vi "Configure System Mode.vi"(8 "error in (no error)":errorcluster, 10 "System Mode (0: Local)":i32(ring) items=["Local", "Remote", "Remote with Lock", "Voltage", "Current", "Dual"], 11 "VISA resource name":refnum<visa-resource-name>) -> (0 "error out":errorcluster, 3 "VISA resource name out":refnum<visa-resource-name>)   [LabVIEW 2018, in "XP Power PLS600.lvlib"]
doc: "Sets the Control Source of the power supply to the specified value. Control Sources include: Local control from the front panel of the instrument, Remote control over the SCPI interface with limited front panel functionality, Remote with Lock control over the SCPI interface with no front panel capability, Analog Voltage Control where the voltage setpoint is determined by the analog voltage input, Analog Current Control where the current setpoint is determined by the analog current input, or Dual Analog Control where the voltage and current setpoint are determined by their respective analog inputs."
uses:
  XP Power PLS600.lvlib
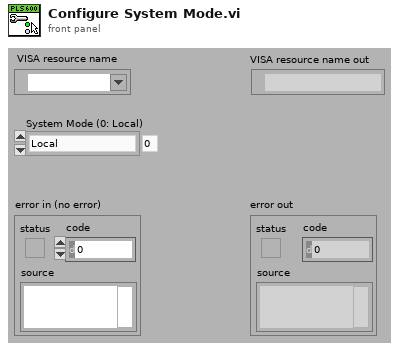
[diagram p1: front panel]
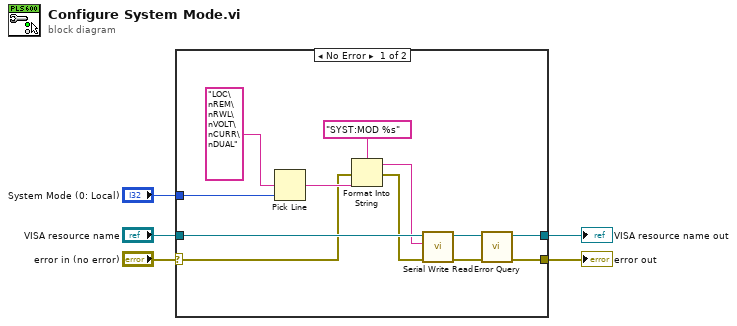
[diagram p0: block diagram]
diagram:
  n1 = case shown="No Error" "error in (no error)" {
    selector: "error in (no error)" -> [w8 w18]
    tunnel: "System Mode (0: Local)" -> [w16 _]
    tunnel: [w15 w19] -> w4
    tunnel: [w14 w18] -> w3
    tunnel: "VISA resource name" -> [w13 w19]
    frame No Error {
      n2 = Pick Line(multi-line string="LOC\nREM\nRWL\nVOLT\nCURR\nDUAL", line index=w16) -> (output string=w9:string)  [unwired: 1 in]
      n3 = Format Into String(format string="SYST:MOD %s" ("Command to Send"), error in=w8, w9) -> (resulting string=w6:string, error out=w7:errorcluster)  [unwired: 1 in]
      n4 = call "Serial Write Read.vi"("error in (no error)"=w7, "Write Buffer"=w6, "VISA resource name"=w13) -> ("error out"=w11:errorcluster, "VISA resource name out"=w12:refnum<visa-resource-name>)  [unwired: 6 in, 1 out]
      n5 = call "Error Query.vi"("error in (no error)"=w11, "VISA resource name"=w12) -> ("error out"=w14:errorcluster, "VISA resource name out"=w15:refnum<visa-resource-name>)  [unwired: 6 in, 2 out]
    }
    frame Error {
    }
  }
  "VISA resource name out" <- w4
  "error out" <- w3
